vi "Concatenate Arrays.vi"(4 "JSON Datatypes":refnum<class "JSON Helper.lvclass">[](array[class]), 5 "JSON Array in":refnum<class "JSON Helper.lvclass">) -> (1 "JSON Array out":refnum<class "JSON Helper.lvclass">)   [LabVIEW 2016, in "JSON Helper.lvclass"]
doc: "Adds multiple elements to the end of a JSON Array"
uses:
  JSON Helper/JSON Helper.lvclass
  JSON Helper/JSON Helper.lvclass/JSON Helper.ctl
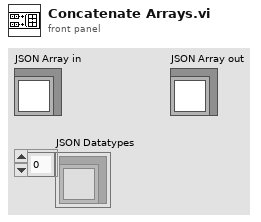
[diagram p1: front panel]
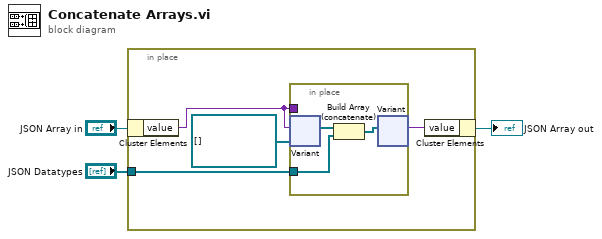
[diagram p0: block diagram]
diagram:
  n1 = in-place {
    in-place-border: "JSON Datatypes" -> [w7]
    n2 = in-place-cluster #1("JSON Array in") -> ("value"=w5:variant)
    n3 = in-place {
      in-place-border: w7 -> [w10]
      in-place-border: w5 -> [_]
      n4 = in-place-variant #2(w5, refnum<class "JSON Helper.lvclass">[] [] ("JSON Datatypes")) -> (w9:refnum<class "JSON Helper.lvclass">[])  [unwired: 1 out]
      n5 = Build Array (concatenate)(w9, w10) -> (w8:refnum<class "JSON Helper.lvclass">[])
      n6 = in-place-variant #2(w8) -> (w4:variant)  [unwired: 1 out]
    }
    n7 = in-place-cluster #1("value"=w4) -> (→"JSON Array out":refnum<class "JSON Helper.lvclass">)
  }
